vi "Partition_Setup.vi"(8 "error in (no error)":errorcluster, 11 "DataCluster in":T1={"Core"={"Current VI Reference"=refnum, "Close Panel on Exit?"=FALSE, "Exit"=FALSE}, "Connections"={"cDAQ Therm"={"Task"="ThermTask", "Connected"=FALSE, "Active"=FALSE}, "cDAQ Voltage"={"Task"="", "Connected"=FALSE, "Active"=FALSE}, "Camera"={"Session"="", "Connected"=FALSE, "Active"=FALSE}}, "Data Acquisition"={"Setup"={"Label"="_41", "Operator"="", "Notes"="", "TempGrad"=1.0, "TargetTemp"=-20.0, "Sample Volume"=1.0}, "Camera"={"Image"=refnum, "Save Image"=refnum}, "Thermistor"={"Sample Size"=5, "Calibration"={"B0.100"=[3450.0, 3450.0, 3450.0, 3450.0, 3450.0, 3450.0, 3450.0, 3450.0], "R25"=[10.74, 10.74, 10.74, 10.74, 10.74, 10.74, 10.74, 10.74], "V_S"=10.0, "R_S"=10.0}, "Timing Mode"=14713}, "Queue"={"Size"=5, "Queue"=refnum}, "Sample Rate"=240, "Active"=FALSE, "Ready"=FALSE, "Partition"={"Data"=[], "Cell Label"="", "Cell Color"=0, "Height"=10, "Width"=16, "Grid"=[]}}, "Control"={"Sample Rate"=20, "PID gains"={"proportional gain (Kc)"=1.0, "integral time (Ti, min)"=0.01, "derivative time (Td, min)"=0.0}}} {"Control"."PID gains"."derivative time (Td, min)" format="%.3f"; "Control"."PID gains"."integral time (Ti, min)" format="%.3f"; "Control"."PID gains"."proportional gain (Kc)" format="%.3f"; "Control"."Sample Rate" min=1 max=20 step=1 format="%.0f Samples/sec"; "Data Acquisition"."Thermistor"."Timing Mode" items=["Automatic"=16097, "High Resolution"=10195, "High Speed"=14712, "Best 50 Hz Rejection"=14713, "Best 60 Hz Rejection"=14714, "Custom"=10137]; "Data Acquisition"."Thermistor"."Calibration"."R_S" min=0.1 max=1000.0 format="%#_g kOhm"; "Data Acquisition"."Thermistor"."Calibration"."V_S" min=5.0 max=48.0 format="%#_g V"; "Data Acquisition"."Thermistor"."Calibration"."R25" min=0.1 max=1000.0 format="%#_g kOhm"; "Data Acquisition"."Thermistor"."Calibration"."B0.100" min=100.0 max=10000.0 format="%#_g K"; "Data Acquisition"."Thermistor"."Sample Size" min=1 max=200; "Data Acquisition"."Sample Rate" min=20 max=240 format="%.0f samples/min"; "Data Acquisition"."Queue"."Size" min=1 max=200; "Data Acquisition"."Setup"."Sample Volume" min=0.0 max=500.0 format="%#_g µL"; "Data Acquisition"."Setup"."TargetTemp" min=-30.0 max=30.0 step=0.5 format="%#_g °C"; "Data Acquisition"."Setup"."TempGrad" min=-100.0 max=100.0 step=0.1 format="%#_g °C/min"}) -> (0 "error out":errorcluster, 3 "DataCluster out":T1={"Core"={"Current VI Reference"=refnum, "Close Panel on Exit?"=FALSE, "Exit"=FALSE}, "Connections"={"cDAQ Therm"={"Task"="ThermTask", "Connected"=FALSE, "Active"=FALSE}, "cDAQ Voltage"={"Task"="", "Connected"=FALSE, "Active"=FALSE}, "Camera"={"Session"="", "Connected"=FALSE, "Active"=FALSE}}, "Data Acquisition"={"Setup"={"Label"="_41", "Operator"="", "Notes"="", "TempGrad"=1.0, "TargetTemp"=-20.0, "Sample Volume"=1.0}, "Camera"={"Image"=refnum, "Save Image"=refnum}, "Thermistor"={"Sample Size"=5, "Calibration"={"B0.100"=[3450.0, 3450.0, 3450.0, 3450.0, 3450.0, 3450.0, 3450.0, 3450.0], "R25"=[10.74, 10.74, 10.74, 10.74, 10.74, 10.74, 10.74, 10.74], "V_S"=10.0, "R_S"=10.0}, "Timing Mode"=14713}, "Queue"={"Size"=5, "Queue"=refnum}, "Sample Rate"=240, "Active"=FALSE, "Ready"=FALSE, "Partition"={"Data"=[["A", "20%", "", "", ""], ["B", "30", "", "", ""], ["C", "5%", "", "", ""], ["D", "35%", "", "", ""], ["E", "...", "", "", ""], ["F", "...", "", "", ""], ["G", "...", "", "", ""], ["X", "Empty", "", "", ""]], "Cell Label"="A", "Cell Color"=29373, "Height"=8, "Width"=12, "Grid"=[["X", "X", "X", "X", "X", "X", "X", "X", "X", "X", "X", "X"], ["X", "X", "X", "X", "X", "X", "X", "X", "X", "X", "X", "X"], ["X", "X", "X", "X", "X", "X", "X", "X", "X", "X", "X", "X"], ["X", "X", "X", "X", "X", "X", "X", "X", "X", "X", "X", "X"], ["X", "X", "X", "X", "X", "X", "X", "X", "X", "X", "X", "X"], ["X", "X", "X", "X", "X", "X", "X", "X", "X", "X", "X", "X"], ["X", "X", "X", "X", "X", "X", "X", "X", "X", "X", "X", "X"], ["X", "X", "X", "X", "X", "X", "X", "X", "X", "X", "X", "X"]]}}, "Control"={"Sample Rate"=20, "PID gains"={"proportional gain (Kc)"=1.0, "integral time (Ti, min)"=0.01, "derivative time (Td, min)"=0.0}}} {"Control"."PID gains"."derivative time (Td, min)" format="%.3f"; "Control"."PID gains"."integral time (Ti, min)" format="%.3f"; "Control"."PID gains"."proportional gain (Kc)" format="%.3f"; "Control"."Sample Rate" min=1 max=20 step=1 format="%.0f Samples/sec"; "Data Acquisition"."Thermistor"."Timing Mode" items=["Automatic"=16097, "High Resolution"=10195, "High Speed"=14712, "Best 50 Hz Rejection"=14713, "Best 60 Hz Rejection"=14714, "Custom"=10137]; "Data Acquisition"."Thermistor"."Calibration"."R_S" min=0.1 max=1000.0 format="%#_g kOhm"; "Data Acquisition"."Thermistor"."Calibration"."V_S" min=5.0 max=48.0 format="%#_g V"; "Data Acquisition"."Thermistor"."Calibration"."R25" min=0.1 max=1000.0 format="%#_g kOhm"; "Data Acquisition"."Thermistor"."Calibration"."B0.100" min=100.0 max=10000.0 format="%#_g K"; "Data Acquisition"."Thermistor"."Sample Size" min=1 max=200; "Data Acquisition"."Sample Rate" min=20 max=240 format="%.0f samples/min"; "Data Acquisition"."Queue"."Size" min=1 max=200; "Data Acquisition"."Setup"."Sample Volume" min=0.0 max=500.0 format="%#_g µL"; "Data Acquisition"."Setup"."TargetTemp" min=-30.0 max=30.0 step=0.5 format="%#_g °C"; "Data Acquisition"."Setup"."TempGrad" min=-100.0 max=100.0 step=0.1 format="%#_g °C/min"})   [LabVIEW 2020]
uses:
  DataCluster.ctl
  <vilib>/userDefined/High Color/IMAQdx.ctl
  <vilib>/vision/Image Controls.llb/IMAQ Image.ctl
  <vilib>/Utility/miscctls.llb/LVRowAndColumnTypeDef.ctl
  <vilib>/Utility/miscctls.llb/LVBoundsTypeDef.ctl
  <vilib>/Utility/xml.llb/Write to XML File(string).vi
  <vilib>/Utility/xml.llb/Read From XML File(string).vi
panel:
  out "Grid":string[][](table)=[["X", "X", "X", "X", "X", "X", "X", "X", "X", "X", "X", "X"], ["X", "X", "X", "X", "X", "X", "X", "X", "X", "X", "X", "X"], ["X", "X", "X", "X", "X", "X", "X", "X", "X", "X", "X", "X"], ["X", "X", "X", "X", "X", "X", "X", "X", "X", "X", "X", "X"], ["X", "X", "X", "X", "X", "X", "X", "X", "X", "X", "X", "X"], ["X", "X", "X", "X", "X", "X", "X", "X", "X", "X", "X", "X"], ["X", "X", "X", "X", "X", "X", "X", "X", "X", "X", "X", "X"], ["X", "X", "X", "X", "X", "X", "X", "X", "X", "X", "X", "X"]]
  in  "Cancel":bool
  in  "OK":bool
  in  "Partition Size":enum32{"12x8", "24x16"}(radio)
  in  "Partitions":i32[](listbox)=[0]
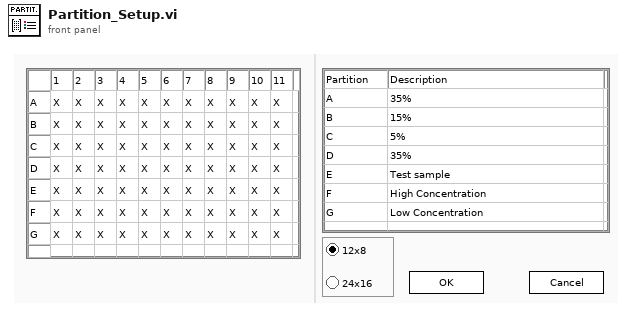
[diagram p1: front panel]
types:
  T1 = typedef "DataCluster.ctl" = cluster{"Core":cluster{"Current VI Reference":refnum<vi>, "Close Panel on Exit?":bool, "Exit":bool}, "Connections":cluster{"cDAQ Therm":cluster{"Task":refnum<k21>, "Connected":bool, "Active":bool}, "cDAQ Voltage":cluster{"Task":refnum<k21>, "Connected":bool, "Active":bool}, "Camera":cluster{"Session":T2, "Connected":bool, "Active":bool}}, "Data Acquisition":cluster{"Setup":cluster{"Label":string, "Operator":string, "Notes":string, "TempGrad":dbl, "TargetTemp":dbl, "Sample Volume":dbl}, "Camera":cluster{"Image":T3, "Save Image":T3}, "Thermistor":cluster{"Sample Size":i32, "Calibration":cluster{"B0.100":dbl[], "R25":dbl[], "V_S":dbl, "R_S":dbl}, "Timing Mode":i32}, "Queue":cluster{"Size":i32, "Queue":refnum<queue>}, "Sample Rate":i32, "Active":bool, "Ready":bool, "Partition":cluster{"Data":string[][], "Cell Label":string, "Cell Color":u32, "Height":i32, "Width":i32, "Grid":string[][]}}, "Control":cluster{"Sample Rate":i32, "PID gains":cluster{"proportional gain (Kc)":dbl, "integral time (Ti, min)":dbl, "derivative time (Td, min)":dbl}}}
  T2 = typedef "IMAQdx.ctl" = refnum<k21>
  T3 = typedef "IMAQ Image.ctl" = refnum<image>
  T4 = typedef "LVRowAndColumnTypeDef.ctl" = cluster{"Row":i32, "Column":i32}
  T5 = cluster{"Data":string[][], "Cell Label":string, "Cell Color":u32, "Height":i32, "Width":i32, "Grid":string[][]}
  T6 = typedef "LVBoundsTypeDef.ctl" = cluster{"Width":u32, "Height":u32}
  T7 = typedef "LVRectTypeDef.ctl" = cluster{"Left":i16, "Top":i16, "Right":i16, "Bottom":i16}
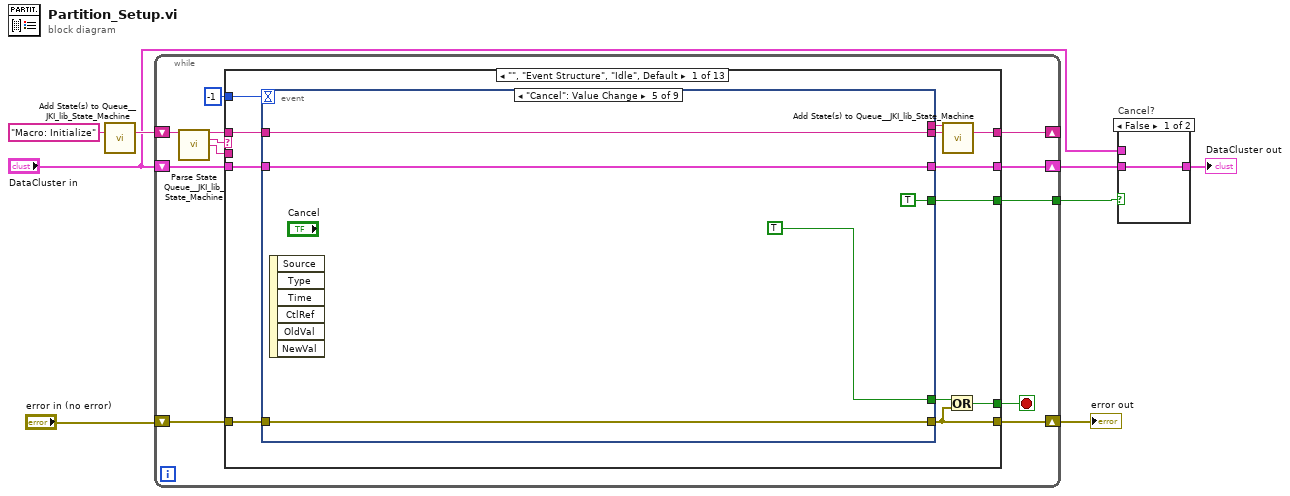
[diagram p0: block diagram]
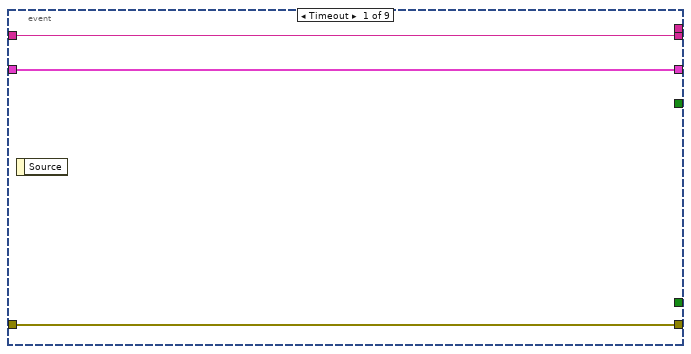
[diagram p3: hidden frame]
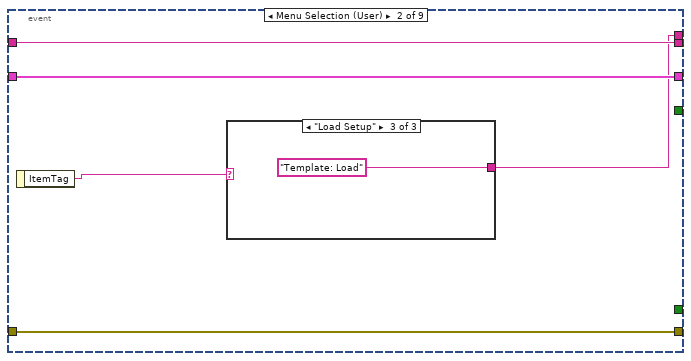
[diagram p4: hidden frame]
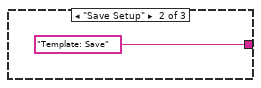
[diagram p6: hidden frame]
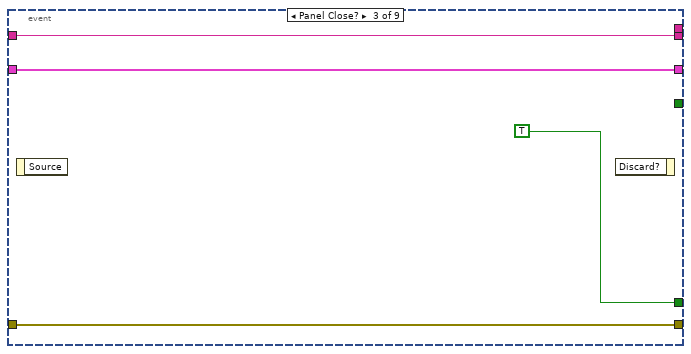
[diagram p7: hidden frame]
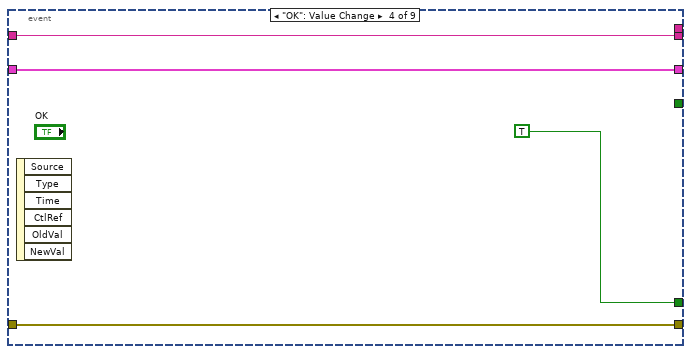
[diagram p8: hidden frame]
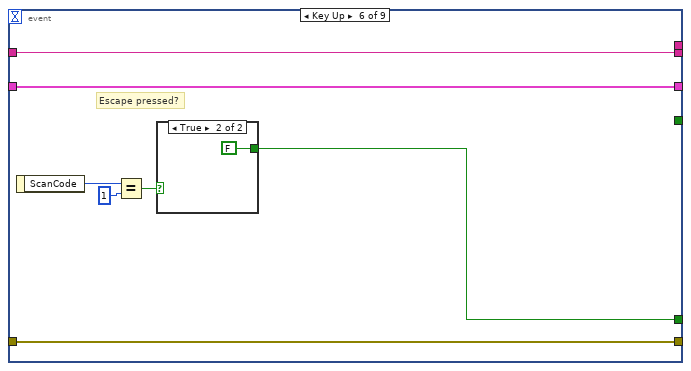
[diagram p9: hidden frame]
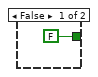
[diagram p10: hidden frame]
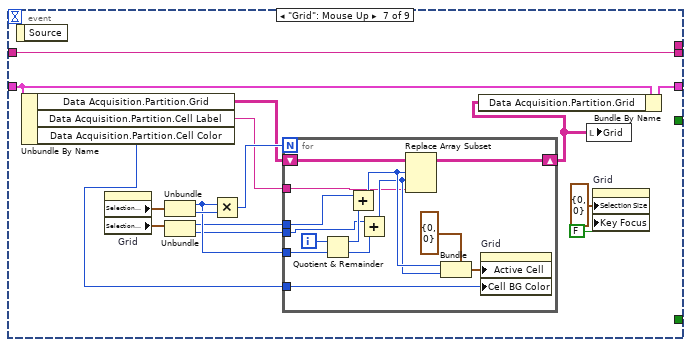
[diagram p11: hidden frame]
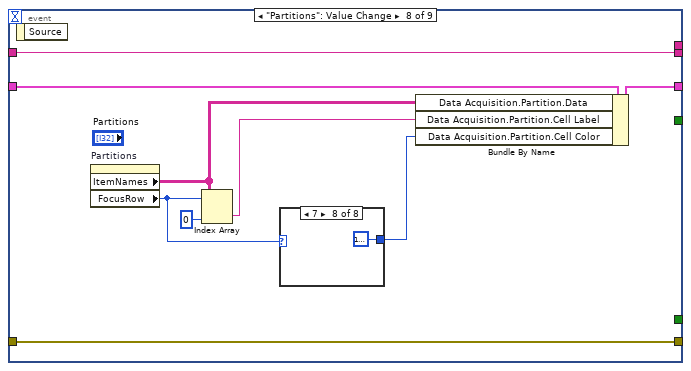
[diagram p12: hidden frame]
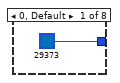
[diagram p13: hidden frame]
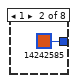
[diagram p14: hidden frame]
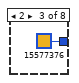
[diagram p15: hidden frame]
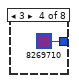
[diagram p16: hidden frame]
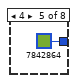
[diagram p17: hidden frame]
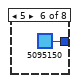
[diagram p18: hidden frame]
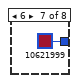
[diagram p19: hidden frame]
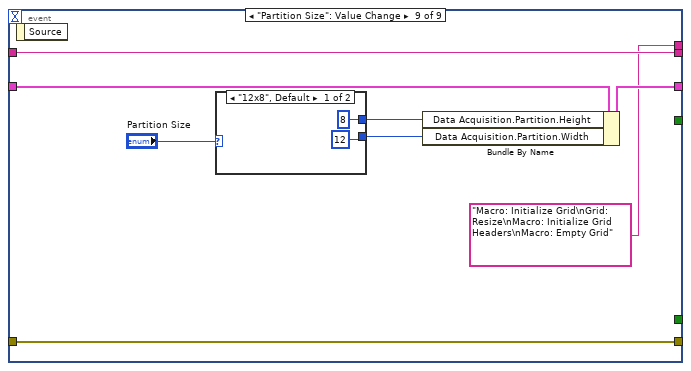
[diagram p20: hidden frame]
diagram:
  n1 = call <vilib>:"Add State(s) to Queue__JKI_lib_State_Machine.vi"("State(s) in (\"\")"="Macro: Initialize") -> ("States Out"=w5:string)  [unwired: 14 in]
  n2 = while {
    shift-right: [w20] -> w3
    shift-left: "DataCluster in" -> [w19]
    shift-right: [w15] -> w8
    shift-left: "error in (no error)" -> [w16]
    shift-right: [w10] -> _
    shift-left: w5 -> [w14]
    tunnel: [w9] -> w2
    stop <- w17 stop-if-true
    n3 = call <vilib>:"Parse State Queue__JKI_lib_State_Machine.vi"("State Queue"=w14) -> ("Remaining States"=w11:string, "Current State"=w13:string, "Arguments"=w12:string)  [unwired: 12 in]
    n4 = case shown="\"\", \"Event Structure\", \"Idle\", Default" w13 {
      tunnel: [w32 w126 w143 w158 w187 w215 w220 w228 w245 w249 w264 w294 w326] -> w20
      tunnel: w19 -> [w31 w126 w143 w157 w187 w215 w220 w224 w245 w249 w264 w298 w326]
      tunnel: -1 -> [w29 _ _ _ _ _ _ _ _ _ _ _ _]
      tunnel: [w28 _ _ _ _ _ _ _ _ _ _ _ _] -> w17
      tunnel: w16 -> [w27 w127 w147 w175 w193 w216 w221 w231 w248 w254 w267 w302 w335]
      tunnel: [w26 w127 w147 w175 w193 w216 w221 w231 w248 w254 w267 w302 w335] -> w15
      tunnel: w12 -> [_ _ _ _ _ _ _ _ _ _ _ _ _]
      tunnel: w11 -> [w25 w124 w145 w173 w191 w213 w218 w229 w246 w252 w265 w300 w333]
      tunnel: [w23 w125 w146 w174 w192 w214 w219 w230 w247 w253 w266 w301 w334] -> w10
      tunnel: [w21 _ _ _ _ _ _ _ _ _ _ _ _] -> w9
      frame "", "Event Structure", "Idle", Default {
        n5 = event shown="[4] \"Cancel\": Value Change" {
          selector: _ -> [_ _ _ _ _ _ _ _ _]
          dyn-events: _ -> [_ _ _ _ _ _ _ _ _]
          timeout: w29 -> [_ _ _ _ _ _ _ _ _]
          tunnel: w31 -> [w33 w39 w44 w48 w53 w57 w71 w103 w119]
          tunnel: [w33 w39 w44 w48 w53 w57 w68 w100 w118] -> w32
          tunnel: [_ _ TRUE TRUE TRUE w62 _ _ _] -> w30
          tunnel: [w35 w40 w45 w49 w54 w58 _ w98 w116] -> w26
          tunnel: w27 -> [w35 w40 w45 w49 w54 w58 _ w98 w116]
          tunnel: [w34 w38 w43 w47 w52 w56 w72 w99 w117] -> w24
          tunnel: w25 -> [w34 w38 w43 w47 w52 w56 w72 w99 w117]
          tunnel: [_ w37 _ _ _ _ _ _ "Macro: Initialize Grid\nGrid: Resize\nMacro: Initialize Grid Headers\nMacro: Empty Grid" ("State(s) in Front (\"\")")] -> w22
          tunnel: [_ _ _ _ TRUE _ _ _ _] -> w21
          event Timeout {
            n6 = event-data() -> ()  [unwired: 1 in, 1 out]
          }
          event Menu Selection (User) {
            n7 = event-data() -> ("ItemTag"=w36:string)  [unwired: 1 in]
            n8 = case shown="\"Load Setup\"" w36 {
              tunnel: [_ "Template: Save" "Template: Load"] -> w37
              frame "False", Default {
              }
              frame "Save Setup" {
              }
              frame "Load Setup" {
              }
            }
          }
          event Panel Close? {
            n9 = event-data() -> ()  [unwired: 1 in, 1 out]
            n10 = event-data() -> ()  [unwired: 2 in, 1 out]
          }
          event "OK": Value Change {
            n11 = event-data() -> ()  [unwired: 1 in, 6 out]
          }
          event "Cancel": Value Change {
            n12 = event-data() -> ()  [unwired: 1 in, 6 out]
          }
          event Key Up {
            # "Escape pressed?"
            n13 = event-data() -> ("ScanCode"=w61:i16)  [unwired: 1 in]
            n14 = Equal?(x=w61, y=i16 1) -> (x = y?=w59:bool)
            n15 = case shown="True" w59 {
              tunnel: [FALSE FALSE] -> w62
              frame False {
              }
              frame True {
              }
            }
          }
          event "Grid": Mouse Up {
            n16 = event-data() -> ()  [unwired: 1 in, 1 out]
            n17 = Unbundle By Name(w71) -> ("Data Acquisition.Partition.Grid"=w66:string[][], "Data Acquisition.Partition.Cell Label"=w70:string, "Data Acquisition.Partition.Cell Color"=w69:u32)
            n18 = property on="Grid" class="Tbl (strict)"() -> ("Selection Size"=w79:T4, "Selection Start"=w76:T4)  [unwired: 2 in, 2 out]
            n19 = Unbundle(w79) -> ("Row"=w77:i32, "Column"=w78:i32)
            n20 = Unbundle(w76) -> ("Row"=w75:i32, "Column"=w74:i32)
            n21 = Multiply(x=w77, y=w78) -> (x*y=w80:i32)
            n22 = for {
              N: w80 -> [_]
              tunnel: w77 -> [w94]
              shift-right: [w90] -> w67
              shift-left: w66 -> [w81]
              tunnel: w75 -> [w89]
              tunnel: w74 -> [w88]
              tunnel: w70 -> [w83]
              tunnel: w69 -> [w82]
              i -> [w93]
              n23 = Quotient & Remainder(x=w93, y=w94) -> (x-y*floor(x/y)=w92:i32, floor(x/y)=w91:i32)
              n24 = Add(x=w89, y=w92) -> (x+y=w85:i32)
              n25 = Add(x=w88, y=w91) -> (x+y=w84:i32)
              n26 = Replace Array Subset(array=w81, new element=w83, index (row)=w85, index (col)=w84) -> (w90:string[][])
              n27 = Bundle(cluster=T4 {"Row"=0, "Column"=0} ("Active Cell:Active Cell"), "Row"=w85, "Column"=w84) -> (w86:T4)
              n28 = property on="Grid" class="Tbl (strict)"("Active Cell"=w86, "Cell BG Color"=w82) -> ()  [unwired: 2 in, 2 out]
            }
            n29 = Bundle By Name(cluster=w71, "Data Acquisition.Partition.Grid"=w67) -> (w68:T1)
            n30 = local write "Grid"(w67) -> ()
            n31 = property on="Grid" class="Tbl (strict)"("Selection Size"=T4 {"Row"=0, "Column"=0} ("Selection Start"), "Key Focus"=FALSE) -> ()  [unwired: 2 in, 2 out]
          }
          event "Partitions": Value Change {
            n32 = event-data() -> ()  [unwired: 1 in, 1 out]
            n33 = property on="Partitions" class="MCListbox (strict)"() -> ("ItemNames"=w95:string[][], "FocusRow"=w101:i32)  [unwired: 2 in, 2 out]
            n34 = Index Array(array=w95, index (row)=w101, index (col)=0 ("disabled index (col)")) -> (element=w97:string)
            n35 = case shown="7" w101 {
              tunnel: [u32 29373 ("Active Cell:Cell Background Color") u32 14242585 ("Active Cell:Cell Background Color") u32 15577376 ("Active Cell:Cell Background Color") u32 8269710 ("Active Cell:Cell Background Color") u32 7842864 ("Active Cell:Cell Background Color") u32 5095150 ("Active Cell:Cell Background Color") u32 10621999 ("Active Cell:Cell Background Color") u32 16777216 ("Active Cell:Cell Background Color")] -> w96
              frame 0, Default {
              }
              frame 1 {
              }
              frame 2 {
              }
              frame 3 {
              }
              frame 4 {
              }
              frame 5 {
              }
              frame 6 {
              }
              frame 7 {
              }
            }
            n36 = Bundle By Name(cluster=w103, "Data Acquisition.Partition.Data"=w95, "Data Acquisition.Partition.Cell Label"=w97, "Data Acquisition.Partition.Cell Color"=w96) -> (w100:T1)
          }
          event "Partition Size": Value Change {
            n37 = event-data() -> ()  [unwired: 1 in, 1 out]
            n38 = case shown="\"12x8\", Default" "Partition Size" {
              tunnel: [8 ("Data Acquisition.Partition.Height") 16 ("Data Acquisition.Partition.Height")] -> w114
              tunnel: [12 ("Data Acquisition.Partition.Width") 24 ("Data Acquisition.Partition.Width")] -> w113
              frame "12x8", Default {
              }
              frame "24x16" {
              }
            }
            n39 = Bundle By Name(cluster=w119, "Data Acquisition.Partition.Height"=w114, "Data Acquisition.Partition.Width"=w113) -> (w118:T1)
          }
        }
        n40 = call <vilib>:"Add State(s) to Queue__JKI_lib_State_Machine.vi"("State(s) in Front (\"\")"=w22, "State(s) in (\"\")"=w24) -> ("States Out"=w23:string)  [unwired: 13 in]
        n41 = Or(x=w30, y=w26) -> (x .or. y?=w28:bool)
      }
      frame "---------- Template ----------" {
        n42 = call <vilib>:"Add State(s) to Queue__JKI_lib_State_Machine.vi"("State(s) in (\"\")"=w124) -> ("States Out"=w125:string)  [unwired: 14 in]
      }
      frame "Template: Save" {
        n43 = call <vilib>:"Application Directory.vi"() -> ("Application Directory"=w139:path)
        n44 = Build Path(base path=w139, name or relative path=path "Partitions") -> (appended path=w140:path)
        n45 = call <vilib>:"Check if File or Folder Exists.vi"("path"=w140) -> ("file or folder exists?"=w142:bool, "dup path"=w141:path)  [unwired: 8 in, 1 out]
        n46 = case shown="False" w142 {
          tunnel: w141 -> [w149 w150]
          tunnel: [w148 w150] -> w133
          frame False {
            n47 = Create Folder(path (use dialog)=w149) -> (created path=w148:path)  [unwired: 2 in, 2 out]
          }
          frame True {
          }
        }
        n48 = Unbundle By Name(w143) -> ("Data Acquisition.Partition"=w144:T5)
        n49 = call "File Dialog3"("start path"=w133, "prompt"="Save Parition Tempalte", "button label"="Save Template", "default name"="Partition Setup", "pattern (all files)"="*.prt", "pattern label"="Partition Template") -> ("selected path"=w136:path, "cancelled"=w134:bool, "error out"=w135:errorcluster)  [unwired: 6 in, 1 out]
        n50 = Or(x=w134, y=w135) -> (x .or. y?=w137:bool)
        n51 = case shown="False" w137 {
          tunnel: w144 -> [w153 _]
          tunnel: w136 -> [w151 _]
          frame False {
            n52 = Flatten To XML(6:w153) -> (2:w152:string)
            n53 = call-poly <vilib>:"Write to XML File.vi"("XML Input"=w152, "XML File Path"=w151) -> ()  [unwired: 7 in, 3 out]
          }
          frame True {
          }
        }
        n54 = call <vilib>:"Add State(s) to Queue__JKI_lib_State_Machine.vi"("State(s) in (\"\")"=w145) -> ("States Out"=w146:string)  [unwired: 14 in]
      }
      frame "Template: Load" {
        n55 = call <vilib>:"Application Directory.vi"() -> ("Application Directory"=w167:path)
        n56 = Build Path(base path=w167, name or relative path=path "Partitions") -> (appended path=w168:path)
        n57 = call <vilib>:"Check if File or Folder Exists.vi"("path"=w168) -> ("file or folder exists?"=w170:bool, "dup path"=w169:path)  [unwired: 8 in, 1 out]
        n58 = case shown="False" w170 {
          tunnel: w169 -> [w177 w178]
          tunnel: [w176 w178] -> w171
          frame False {
            n59 = Create Folder(path (use dialog)=w177) -> (created path=w176:path)  [unwired: 2 in, 2 out]
          }
          frame True {
          }
        }
        n60 = Unbundle By Name(w157) -> ("Data Acquisition.Partition"=w172:T5)
        n61 = call "File Dialog2"("start path"=w171, "prompt"="Load Parition Tempalte", "button label"="Load Template", "default name"="Partition Setup", "pattern (all files)"="*.prt", "pattern label"="Partition Template") -> ("selected path"=w160:path, "cancelled"=w159:bool)  [unwired: 6 in, 2 out]
        n62 = case shown="False" w159 {
          tunnel: w172 -> [w181 w183]
          tunnel: w160 -> [w182 _]
          tunnel: [w179 w183] -> w155
          frame False {
            n63 = call-poly <vilib>:"Read From XML File.vi"("XML File Path"=w182) -> ("XML Elements"=w180:string)  [unwired: 8 in, 2 out]
            n64 = Unflatten From XML(xml string=w180, type=w181) -> (value=w179:T5)  [unwired: 1 in, 1 out]
          }
          frame True {
          }
        }
        n65 = Bundle By Name(cluster=w157, "Data Acquisition.Partition"=w155) -> (w158:T1)
        n66 = Unbundle By Name(w155) -> ("Grid"=w154:string[][])
        n67 = local write "Grid"(w154) -> ()
        n68 = call <vilib>:"Add State(s) to Queue__JKI_lib_State_Machine.vi"("State(s) in Front (\"\")"="Grid: Resize\nMacro: Initialize Grid Headers\nTemplate: Apply" ("State(s) in Front (\"\")"), "State(s) in (\"\")"=w173) -> ("States Out"=w174:string)  [unwired: 13 in]
      }
      frame "Template: Apply" {
        n69 = Unbundle By Name(w187) -> ("Data Acquisition.Partition.Grid"=w186:string[][], "Data Acquisition.Partition.Data"=w190:string[][], "Data Acquisition.Partition.Height"=w188:i32, "Data Acquisition.Partition.Width"=w185:i32)
        n70 = case shown="12, Default" w185 {
          tunnel: [1 0] -> w184
          frame 24 {
          }
          frame 12, Default {
          }
        }
        n71 = local write "Partition Size"(w184) -> ()
        n72 = Multiply(x=w188, y=w185) -> (x*y=w189:i32)
        n73 = for {
          N: w189 -> [_]
          tunnel: w188 -> [w204]
          tunnel: w186 -> [w200]
          i -> [w203]
          n74 = Quotient & Remainder(x=w203, y=w204) -> (x-y*floor(x/y)=w199:i32, floor(x/y)=w198:i32)
          n75 = Index Array(array=w200, index (row)=w199, index (col)=w198) -> (element=w197:string)
          n76 = case shown="\"X\"" w197 {
            tunnel: [u32 29373 ("Active Cell:Cell Background Color") u32 14242585 ("Active Cell:Cell Background Color") u32 15577376 ("Active Cell:Cell Background Color") u32 8269710 ("Active Cell:Cell Background Color") u32 7842864 ("Active Cell:Cell Background Color") u32 5095150 ("Active Cell:Cell Background Color") u32 10621999 ("Active Cell:Cell Background Color") u32 16777216 ("Active Cell:Cell Background Color")] -> w196
            frame "A", Default {
            }
            frame "B" {
            }
            frame "C" {
            }
            frame "D" {
            }
            frame "E" {
            }
            frame "F" {
            }
            frame "G" {
            }
            frame "X" {
            }
          }
          n77 = Bundle(cluster=T4 {"Row"=0, "Column"=0} ("Active Cell:Active Cell"), "Row"=w199, "Column"=w198) -> (w201:T4)
          n78 = property on="Grid" class="Tbl (strict)"("Active Cell"=w201, "Cell BG Color"=w196) -> ()  [unwired: 2 in, 2 out]
        }
        n79 = property on="Partitions" class="MCListbox (strict)"("ItemNames"=w190) -> ()  [unwired: 2 in, 2 out]
        n80 = call <vilib>:"Add State(s) to Queue__JKI_lib_State_Machine.vi"("State(s) in (\"\")"=w191) -> ("States Out"=w192:string)  [unwired: 14 in]
      }
      frame "---------- Macro ----------" {
        n81 = call <vilib>:"Add State(s) to Queue__JKI_lib_State_Machine.vi"("State(s) in (\"\")"=w213) -> ("States Out"=w214:string)  [unwired: 14 in]
      }
      frame "Macro: Initialize" {
        n82 = call <vilib>:"Add State(s) to Queue__JKI_lib_State_Machine.vi"("State(s) in Front (\"\")"="Macro: Initialize Size\nGrid: Resize\nMacro: Initialize Grid\nMacro: Initialize Grid Headers\nMacro: Initialize Partition Table\nTemplate: Apply" ("State(s) in Front (\"\")"), "State(s) in (\"\")"=w218) -> ("States Out"=w219:string)  [unwired: 13 in]
      }
      frame "Macro: Initialize Partition Table" {
        w222 = T4 {"Row"=0, "Column"=0} ("Selected Cell")
        n83 = for {
          N: 8 -> [_]
          i -> [w233]
          n84 = Bundle(w233, 0) -> (w234:cluster{i32, i32})  [unwired: 1 in]
          n85 = case shown="7" w233 {
            tunnel: [u32 29373 ("Active Cell:Cell Background Color") u32 14242585 ("Active Cell:Cell Background Color") u32 15577376 ("Active Cell:Cell Background Color") u32 8269710 ("Active Cell:Cell Background Color") u32 7842864 ("Active Cell:Cell Background Color") u32 5095150 ("Active Cell:Cell Background Color") u32 10621999 ("Active Cell:Cell Background Color") u32 16777216 ("Active Cell:Cell Background Color")] -> w232
            frame 0, Default {
            }
            frame 1 {
            }
            frame 2 {
            }
            frame 3 {
            }
            frame 4 {
            }
            frame 5 {
            }
            frame 6 {
            }
            frame 7 {
            }
          }
          n86 = property on="Partitions" class="MCListbox (strict)"("ActiveCell"=w234, "CellBG"=w232) -> ()  [unwired: 2 in, 2 out]
        }
        n87 = property on="Partitions" class="MCListbox (strict)"() -> ("ItemNames"=w227:string[][])  [unwired: 2 in, 2 out]
        n88 = Bundle By Name(cluster=w224, "Data Acquisition.Partition.Data"=w227, "Data Acquisition.Partition.Cell Label"="A", "Data Acquisition.Partition.Cell Color"=u32 29373 ("Active Cell:Cell Background Color")) -> (w228:T1)
        n89 = property on="Partitions" class="MCListbox (strict)"("SelectedCell"=w222, "TopLeft"=w222) -> ()  [unwired: 2 in, 2 out]
        n90 = call <vilib>:"Add State(s) to Queue__JKI_lib_State_Machine.vi"("State(s) in (\"\")"=w229) -> ("States Out"=w230:string)  [unwired: 14 in]
      }
      frame "Macro: Initialize Grid" {
        n91 = Unbundle By Name(w245) -> ("Data Acquisition.Partition.Grid"=→"Grid":string[][])
        n92 = call <vilib>:"Add State(s) to Queue__JKI_lib_State_Machine.vi"("State(s) in (\"\")"=w246) -> ("States Out"=w247:string)  [unwired: 14 in]
      }
      frame "Macro: Initialize Size" {
        n93 = Unbundle By Name(w249) -> ("Data Acquisition.Partition.Width"=w250:i32)
        n94 = case shown="12, Default" w250 {
          tunnel: [1 0] -> w251
          frame 24 {
          }
          frame 12, Default {
          }
        }
        n95 = local write "Partition Size"(w251) -> ()
        n96 = call <vilib>:"Add State(s) to Queue__JKI_lib_State_Machine.vi"("State(s) in (\"\")"=w252) -> ("States Out"=w253:string)  [unwired: 14 in]
      }
      frame "Macro: Initialize Grid Headers" {
        n97 = Unbundle By Name(w264) -> ("Data Acquisition.Partition.Width"=w259:i32, "Data Acquisition.Partition.Height"=w258:i32)
        n98 = for {
          N: w259 -> [_]
          shift-right: [w291] -> w262
          shift-left: string[] [] -> [w289]
          i -> [w292]
          n99 = Increment(x=w292) -> (x+1=w288:i32)
          n100 = Number To Decimal String(number=w288) -> (decimal integer string=w290:string)  [unwired: 1 in]
          n101 = Build Array (concatenate)(w289, w290) -> (w291:string[])
        }
        n102 = for {
          N: w258 -> [_]
          shift-right: [w269] -> w263
          shift-left: string[] [] -> [w268]
          i -> [w271]
          n103 = case shown="15" w271 {
            tunnel: ["A" "B" "C" "D" "E" "F" "G" "H" "I" "J" "K" "L" "M" "N" "O" "P"] -> w270
            frame 0, Default {
            }
            frame 1 {
            }
            frame 2 {
            }
            frame 3 {
            }
            frame 4 {
            }
            frame 5 {
            }
            frame 6 {
            }
            frame 7 {
            }
            frame 8 {
            }
            frame 9 {
            }
            frame 10 {
            }
            frame 11 {
            }
            frame 12 {
            }
            frame 13 {
            }
            frame 14 {
            }
            frame 15 {
            }
          }
          n104 = Build Array (concatenate)(w268, w270) -> (w269:string[])
        }
        n105 = property on="Grid" class="Tbl (strict)"("Column Headers[]"=w262, "Row Headers[]"=w263) -> ()  [unwired: 2 in, 2 out]
        n106 = Wait (ms)(milliseconds to wait=u32 20) -> ()  [unwired: 1 out]
        n107 = call <vilib>:"Add State(s) to Queue__JKI_lib_State_Machine.vi"("State(s) in (\"\")"=w265) -> ("States Out"=w266:string)  [unwired: 14 in]
      }
      frame "Macro: Empty Grid" {
        n108 = Unbundle By Name(w298) -> ("Data Acquisition.Partition.Height"=w296:i32, "Data Acquisition.Partition.Width"=w295:i32)
        n109 = Multiply(x=w296, y=w295) -> (x*y=w299:i32)
        n110 = for {
          N: w299 -> [_]
          tunnel: w295 -> [w308]
          i -> [w309]
          (unwired) T6 {"Width"=20, "Height"=20} ("Size")
          n111 = Quotient & Remainder(x=w309, y=w308) -> (x-y*floor(x/y)=w303:i32, floor(x/y)=w304:i32)
          n112 = Bundle(cluster=T4 {"Row"=0, "Column"=0} ("Active Cell:Active Cell"), "Row"=w304, "Column"=w303) -> (w306:T4)
          n113 = property on="Grid" class="Tbl (strict)"("Active Cell"=w306, "Cell BG Color"=u32 16777216 ("Active Cell:Cell Background Color")) -> ()  [unwired: 2 in, 2 out]
        }
        n114 = Initialize Array("X", w296, w295) -> (w293:string[][])
        n115 = Bundle By Name(cluster=w298, "Data Acquisition.Partition.Grid"=w293) -> (w294:T1)
        n116 = local write "Grid"(w293) -> ()
        n117 = call <vilib>:"Add State(s) to Queue__JKI_lib_State_Machine.vi"("State(s) in (\"\")"=w300) -> ("States Out"=w301:string)  [unwired: 14 in]
      }
      frame "Grid: Resize" {
        w327 = 21.18 ("y")
        n118 = Unbundle By Name(w326) -> ("Data Acquisition.Partition.Width"=w328:i32, "Data Acquisition.Partition.Height"=w314:i32)
        n119 = case shown="8" w314 {
          tunnel: [i16 870 i16 620] -> w320
          tunnel: [i16 445 ("y") i16 310 ("y")] -> w316
          frame 24, Default {
          }
          frame 8 {
          }
        }
        n120 = Current VI's Path() -> (path=w324:path)
        n121 = Open VI Reference(vi path=w324) -> (vi reference=w325:refnum<vi>, error out=w313:errorcluster)  [unwired: 5 in]
        n122 = property class="VI"(reference=w325, error in=w313) -> (reference out=w323:refnum<vi>, error out=w312:errorcluster, "Front Panel.WinBounds"=w310:T7)
        n123 = Unbundle By Name(w310) -> ("Left"=w321:i16, "Top"=w318:i16)
        n124 = Increment(x=w328) -> (x+1=w331:i32)
        n125 = Increment(x=w314) -> (x+1=w329:i32)
        n126 = Add(x=w321, y=w320) -> (x+y=w319:i16)
        n127 = Add(x=w318, y=w316) -> (x+y=w317:i16)
        n128 = Multiply(x=w331, y=w327) -> (x*y=w332:dbl)
        n129 = Multiply(x=w329, y=w327) -> (x*y=w330:dbl)
        n130 = Bundle By Name(cluster=w310, "Right"=w319, "Bottom"=w317) -> (w322:T7)
        n131 = property on="Grid" class="Tbl (strict)"("Width"=w332, "Height"=w330) -> ()  [unwired: 2 in, 2 out]
        n132 = property class="VI"(reference=w323, error in=w312, "Front Panel.WinBounds"=w322) -> (reference out=w315:refnum<vi>, error out=w311:errorcluster)
        n133 = Close Reference(reference=w315, error in (no error)=w311) -> ()  [unwired: 1 out]
        n134 = call <vilib>:"Add State(s) to Queue__JKI_lib_State_Machine.vi"("State(s) in (\"\")"=w333) -> ("States Out"=w334:string)  [unwired: 14 in]
      }
    }
  }
  "error out" <- w8
  n135 = case "Cancel?" shown="False" w2 {
    tunnel: [w340 w341] -> w4
    tunnel: w3 -> [w340 _]
    tunnel: "DataCluster in" -> [_ w341]
    frame False {
    }
    frame True {
    }
  }
  "DataCluster out" <- w4
